vi "Log Trace.vi"(8 "error in (no error)":errorcluster, 10 "Trace In":refnum<class "Trace.lvclass">, 11 "Tracer-V in":refnum<class "Tracer-V.lvclass">) -> (0 "error out":errorcluster, 2 "Trace Out":refnum<class "Trace.lvclass">, 3 "Tracer-V out":refnum<class "Tracer-V.lvclass">)   [LabVIEW 2013, in "Tracer-V.lvclass"]
uses:
  Tracer-V.lvclass
  Logical Systems/TraceMessage/Trace.lvclass
  Logical Systems/Tracer/Tracer.lvclass
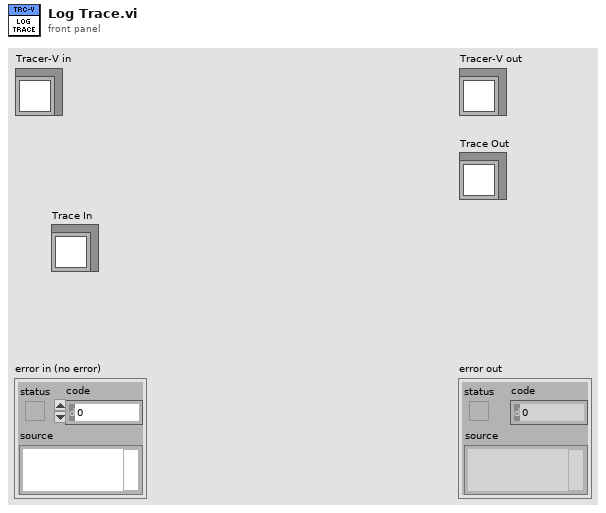
[diagram p1: front panel]
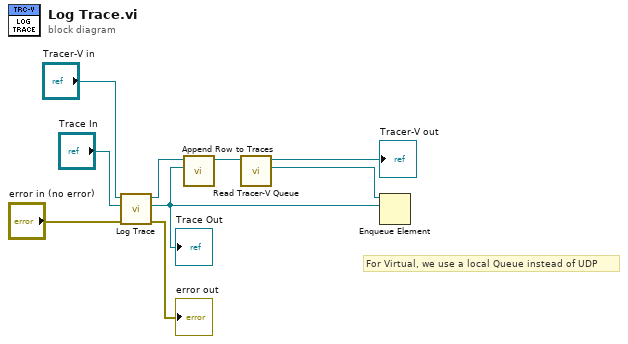
[diagram p0: block diagram]
diagram:
  # "For Virtual, we use a local Queue instead of UDP"
  n1 = call-parent "Log Trace.vi"("error in (no error)"="error in (no error)", "Trace.lvclass"="Trace In", "Tracer in"="Tracer-V in") -> ("error out"=→"error out":errorcluster, "TraceMessage Out"=w1:refnum<class "Trace.lvclass">, "Tracer out"=w2:refnum<class "Tracer-V.lvclass">)  [unwired: 6 in]
  "Trace Out" <- w1
  n2 = call-dynamic "Append Row to Traces.vi"("Trace.lvclass"=w1, "Tracer-V in"=w2) -> ("Tracer-V out"=w4:refnum<class "Tracer-V.lvclass">)  [unwired: 8 in, 1 out]
  n3 = call-dynamic "Read Tracer-V Queue.vi"("Tracer-V in"=w4) -> ("TraceMessage Queue"=w6:refnum<queue>, "Tracer-V out"=→"Tracer-V out":refnum<class "Tracer-V.lvclass">)  [unwired: 8 in, 1 out]
  n4 = Enqueue Element(queue=w6, element=w1) -> ()  [unwired: 2 in, 3 out]
